vi "Prepare - Load and Apply Window Settings - Validate Size.vi"(6 "Minimum":i16, 7 "New Size":i16, 10 "Current Right/Bottom":i16, 11 "Current Left/Top":i16) -> (2 "New Right/Bottom":i16, 3 "New Left/Top":i16)   [LabVIEW 2022 SP3, in "UI Manager.lvlib"]
doc: "____\nHAMPEL SOFTWARE ENGINEERING v2.6.0 (2023-12-19 10:54)"
uses:
  UI Manager.lvlib
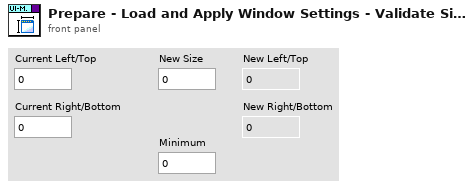
[diagram p1: front panel]
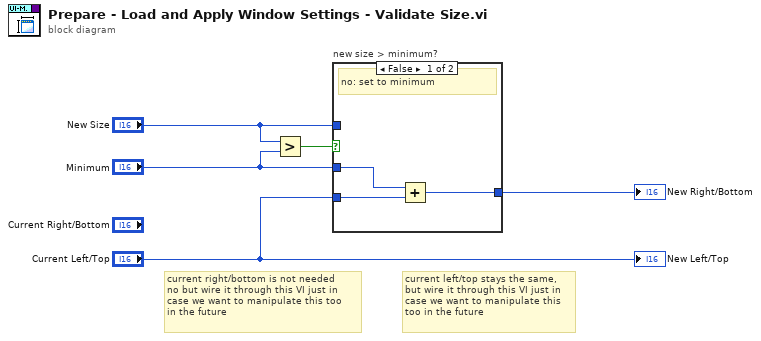
[diagram p0: block diagram]
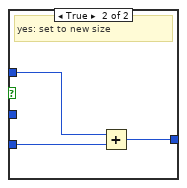
[diagram p2: hidden frame]
diagram:
  # "current right/bottom is not needed\nno but wire it through this VI just in\ncase we want to manipulate this too \nin the future"
  # "current left/top stays the same,\nbut wire it through this VI just in\ncase we want to manipulate this\ntoo in the future"
  n1 = Greater?(x="New Size", y="Minimum") -> (0:w5:bool)
  n2 = case "new size > minimum?" shown="False" w5 {
    tunnel: "New Size" -> [_ w11]
    tunnel: [w6 w10] -> w3
    tunnel: "Minimum" -> [w8 _]
    tunnel: "Current Left/Top" -> [w7 w9]
    frame False {
      # "no: set to minimum"
      n3 = Add(x=w8, y=w7) -> (x+y=w6:i16)
    }
    frame True {
      # "yes: set to new size"
      n4 = Add(x=w11, y=w9) -> (x+y=w10:i16)
    }
  }
  "New Right/Bottom" <- w3
  "New Left/Top" <- "Current Left/Top"
